vi "arm-lift-PID-control.vi"(10 "PV Deg":dbl, 11 "SP DEG":dbl) -> (3 "CO Motor Out":dbl)   [LabVIEW 2019]
uses:
  <vilib>/Rock Robotics/WPI/ThirdParty/JAS_Junk/TrajLib/SlewRateLimiter_New.vi
  <vilib>/Rock Robotics/WPI/ThirdParty/JAS_Junk/TrajLib/SlewRateLimiter_Reset.vi
  <vilib>/Rock Robotics/WPI/ThirdParty/JAS_Junk/TrajLib/SlewRateLimiter_Calculate.vi
  <vilib>/Rock Robotics/WPI/ThirdParty/JAS_Junk/TrajLib/SlewRateLimiter_SetRate.vi
  <vilib>/Rock Robotics/WPI/ThirdParty/JAS_Junk/TrajLib/PIDController_AtSetpoint.vi
  <vilib>/Rock Robotics/WPI/ThirdParty/JAS_Junk/TrajLib/PIDController_SetPIDF.vi
  <vilib>/Rock Robotics/WPI/ThirdParty/JAS_Junk/TrajLib/PIDController_SetDerivativeFilter.vi
  <vilib>/Rock Robotics/WPI/ThirdParty/JAS_Junk/TrajLib/PIDController_SetIntegratorRange.vi
  <vilib>/Rock Robotics/WPI/ThirdParty/JAS_Junk/TrajLib/PIDController_SetTolerancePandV.vi
  <vilib>/Rock Robotics/WPI/ThirdParty/JAS_Junk/TrajLib/PIDController_DisableContinousInput.vi
  <vilib>/Rock Robotics/WPI/ThirdParty/JAS_Junk/TrajLib/PIDController_EnableContinousInput.vi
  <vilib>/Rock Robotics/WPI/ThirdParty/JAS_Junk/TrajLib/PIDController_Reset.vi
  <vilib>/Rock Robotics/WPI/ThirdParty/JAS_Junk/TrajLib/PIDController_New.vi
  <vilib>/Rock Robotics/WPI/ThirdParty/JAS_Junk/TrajLib/PIDController_SetOutputLimits.vi
  <vilib>/Rock Robotics/WPI/ThirdParty/JAS_Junk/TrajLib/Util_GetTime.vi
  <vilib>/Rock Robotics/WPI/ThirdParty/JAS_Junk/TrajLib/PIDController_NewPeriod.vi
  <vilib>/Rock Robotics/WPI/ThirdParty/JAS_Junk/TrajLib/VI/Util_GetTime_U32.vi
  <vilib>/Rock Robotics/SystemInterfaces/NetworkCommunication/NetComm_UsageReport_report.vi
  <vilib>/Rock Robotics/WPI/ThirdParty/JAS_Junk/TrajLib/VI/Util_GetTime_U64.vi
  <vilib>/Rock Robotics/WPI/ThirdParty/JAS_Junk/TrajLib/Globals/Util_LibraryGlobals.vi
  <vilib>/Rock Robotics/WPI/ThirdParty/JAS_Junk/TrajLib/PIDController_AdvCalculate_FF_Sp_Pv.vi
  <vilib>/Rock Robotics/WPI/ThirdParty/JAS_Junk/TrajLib/Trajectory_Library.lvlib
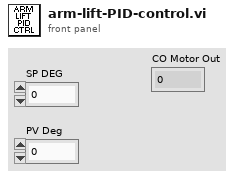
[diagram p1: front panel]
types:
  T1 = typedef "Trajectory_Library.lvlib/PID_ADV_LIMITS.ctl" = cluster{"MaxInput":dbl, "MinInput":dbl, "Continuous":bool, "MaxOutput":dbl, "MinOutput":dbl}
  T2 = typedef "Trajectory_Library.lvlib/PID_ADV_TUNING.ctl" = cluster{"Kf":dbl, "Kp":dbl, "Ki":dbl, "Kd":dbl, "MaximumIntegral":dbl, "MinimumIntegral":dbl, "Filter Derivative":bool}
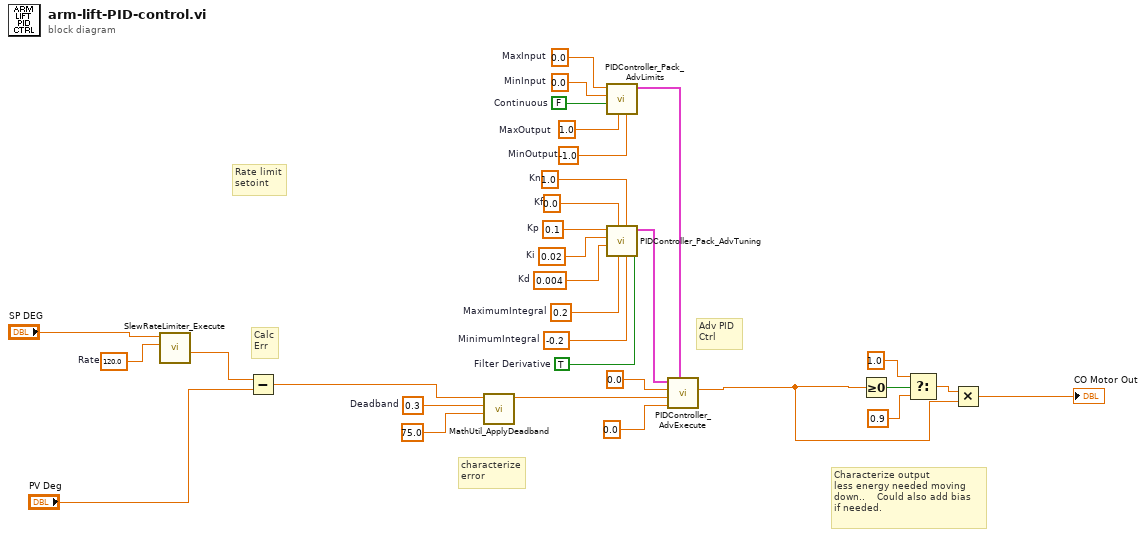
[diagram p0: block diagram]
diagram:
  w24 = 120.0  # Rate
  w22 = 0.3  # Deadband
  w6 = 1.0  # Kn
  w7 = 0.1  # Kp
  w8 = 0.02  # Ki
  w9 = 0.004  # Kd
  w10 = 0.0  # Kf
  w11 = 0.2  # MaximumIntegral
  w12 = -0.2  # MinimumIntegral
  w13 = TRUE  # Filter Derivative
  w15 = 0.0  # MinInput
  w16 = FALSE  # Continuous
  w17 = 1.0  # MaxOutput
  w14 = -1.0  # MinOutput
  w18 = 0.0  # MaxInput
  # "Calc\nErr"
  # "Characterize output\nless energy needed moving\ndown..    Could also add bias\nif needed."
  # "Rate limit\nsetoint"
  # "characterize\nerror"
  # "Adv PID\nCtrl"
  n1 = call <vilib>:"SlewRateLimiter_Execute.vi"("PositiveRate"=w24, "Input"="SP DEG") -> ("Output"=w5:dbl)  [unwired: 8 in, 1 out]
  n2 = Subtract(x=w5, y="PV Deg") -> (x-y=w3:dbl)
  n3 = call <vilib>:"MathUtil_ApplyDeadband.vi"("Max Magnitude"=75.0, "Deadband"=w22, "Value"=w3) -> ("Result"=w1:dbl)  [unwired: 8 in]
  n4 = call <vilib>:"PIDController_Pack_AdvLimits.vi"("MinOutput"=w14, "MaxOutput"=w17, "Continuous"=w16, "MinInput"=w15, "MaxInput"=w18) -> ("Adv PID Limits"=w20:T1)  [unwired: 6 in]
  n5 = call <vilib>:"PIDController_Pack_AdvTuning.vi"("Filter Derivative"=w13, "MinimumIntegral"=w12, "Kn"=w6, "MaximumIntegral"=w11, "Kf"=w10, "Kd"=w9, "Ki"=w8, "Kp"=w7) -> ("Adv PID Tuning"=w19:T2)  [unwired: 3 in]
  n6 = call <vilib>:"PIDController_AdvExecute.vi"("Adv PID Limits"=w20, "FF-FeedForward"=0.0, "SP-SetPoint"=w1, "PV-Measurement"=0.0, "Adv PID Tuning"=w19) -> ("CO-ControlOutput"=w29:dbl)  [unwired: 4 in, 2 out]
  n7 = Greater Or Equal To 0?(x=w29) -> (x >= 0?=w25:bool)
  n8 = Select(t=1.0, s=w25, f=0.9) -> (s? t:f=w28:dbl)
  n9 = Multiply(x=w28, y=w29) -> (x*y=→"CO Motor Out":dbl)
